vi "Destroy.vi"(0 "reference in":refnum<class "Temp.lvclass">, 5 "error in (no error)":errorcluster) -> (14 "reference out":refnum<class "Temp.lvclass">, 19 "error out":errorcluster)   [LabVIEW 2017, in "Temp.lvclass"]
uses:
  Temp.lvclass
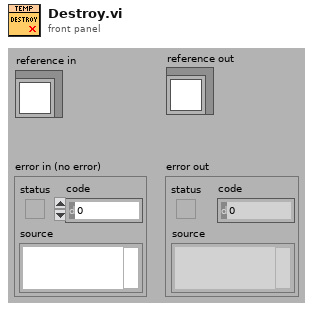
[diagram p1: front panel]
types:
  T1 = typedef "Temp.lvclass/ObjectAttributes.ctl" = cluster{"Temperature Task":refnum<k21>, "Temperature Readings":dbl[], "Thermocouple Type":i32, "Temperature Units":i32, "Average Temperature":dbl, "Number of Temperature Modules":i32, "Number of Total Temperature Channels":i32, "Temperature On/Off Status":bool, "Temperature Module Names (NI-Max Name)":string[], "Number of Channels Per Temperature  Module":i32[], "Temperature VI Reference":refnum<vi>}
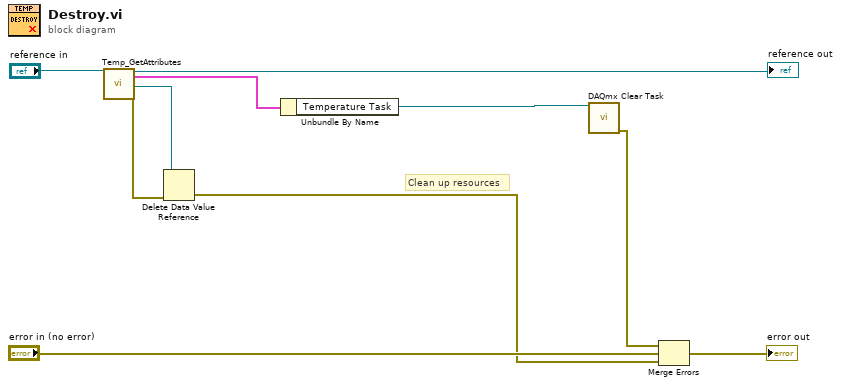
[diagram p0: block diagram]
diagram:
  # "Clean up resources"
  n1 = call "Temp_GetAttributes.vi"("reference in"="reference in") -> ("reference out"=→"reference out":refnum<class "Temp.lvclass">, "Data"=w3:T1, "DataRef"=w6:refnum<data-value>, "error out"=w7:errorcluster)  [unwired: 15 in]
  n2 = Delete Data Value Reference(data value reference=w6, error in=w7) -> (error out=w4:errorcluster)  [unwired: 1 out]
  n3 = Unbundle By Name(w3) -> ("Temperature Task"=w2:refnum<k21>)
  n4 = call <vilib>:"DAQmx Clear Task.vi"("task in"=w2) -> ("error out"=w1:errorcluster)  [unwired: 14 in]
  n5 = Merge Errors(w1, "error in (no error)", w4) -> (→"error out":errorcluster)
